vi "Init DFRobot_Gravity_GNSS.vi"(8 "error in (no error)":errorcluster, 11 "DFRobot_Gravity_GNSS in":refnum<class "DFRobot_Gravity_GNSS.lvclass">) -> (0 "error out":errorcluster, 3 "DFRobot_Gravity_GNSS out":refnum<class "DFRobot_Gravity_GNSS.lvclass">)   [LabVIEW 2020, in "CTI-Peripheral.lvlib" / "DFRobot_Gravity_GNSS.lvclass"]
uses:
  DFRobot_Gravity_GNSS.lvclass
  GPSData.ctl
  Power.ctl
  eGnssMode.ctl
  DFRobot_Gravity_GNSS.lvclass/DFRobot_Gravity_GNSS.ctl
  CTI/I2C Connection/I2C Connection.lvclass/I2C Connection.ctl
  CTI/Session/I2C Write Data.vi
  CTI/I2C Connection/I2C Connection.lvclass
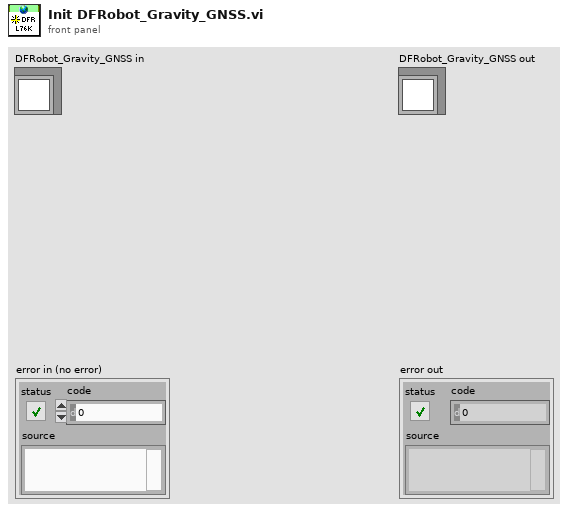
[diagram p1: front panel]
types:
  T1 = typedef "CTI-Peripheral.lvlib/DFRobot_Gravity_GNSS.lvclass/eGnssMode.ctl" = enum16{"No Mode - Error", "eGPS", "eBeiDou", "eGPS_BeiDou", "eGLONASS", "eGPS_eGLONASS", "eGPS_BeiDou_GLONASS"}
  T2 = typedef "CTI-Peripheral.lvlib/DFRobot_Gravity_GNSS.lvclass/GPSData.ctl" = u16
  T3 = typedef "CTI-Peripheral.lvlib/DFRobot_Gravity_GNSS.lvclass/Power.ctl" = enum16{"Enable", "Disable"}
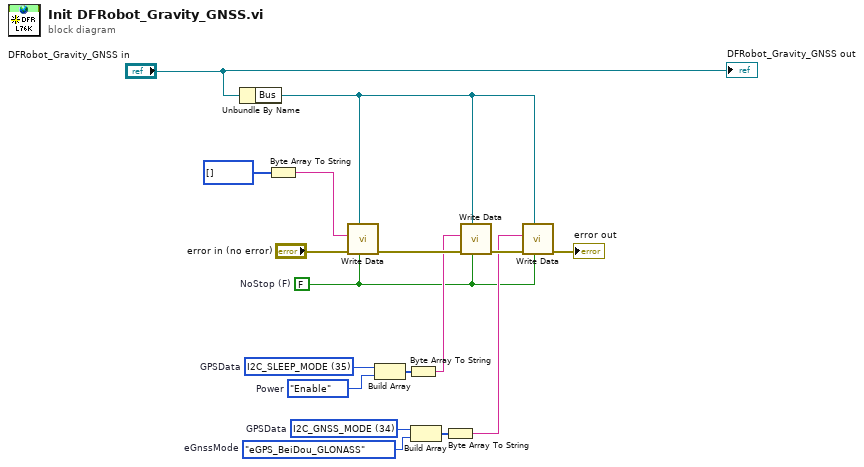
[diagram p0: block diagram]
diagram:
  w2 = eGnssMode."eGPS_BeiDou_GLONASS"  # eGnssMode
  w3 = T2 34 items=["I2C_YEAR_H", "I2C_YEAR_L", "I2C_MONTH", "I2C_DATE", "I2C_HOUR", "I2C_MINUTE", "I2C_SECOND", "I2C_LAT_1", "I2C_LAT_2", "I2C_LAT_X_24", "I2C_LAT_X_16", "I2C_LAT_X_8", "I2C_LON_DIS", "I2C_LON_1", "I2C_LON_2", "I2C_LON_X_24", "I2C_LON_X_16", "I2C_LON_X_8", "I2C_LAT_DIS", "I2C_USE_STAR", "I2C_ALT_H", "I2C_ALT_L", "I2C_ALT_X", "I2C_SOG_H", "I2C_SOG_L", "I2C_SOG_X", "I2C_COG_H", "I2C_COG_L", "I2C_COG_X", "I2C_START_GET", "I2C_ID", "I2C_DATA_LEN_H", "I2C_DATA_LEN_L", "I2C_ALL_DATA", "I2C_GNSS_MODE", "I2C_SLEEP_MODE", "I2C_RGB_MODE"]  # GPSData
  w5 = Power."Enable"  # Power
  w6 = T2 35 items=["I2C_YEAR_H", "I2C_YEAR_L", "I2C_MONTH", "I2C_DATE", "I2C_HOUR", "I2C_MINUTE", "I2C_SECOND", "I2C_LAT_1", "I2C_LAT_2", "I2C_LAT_X_24", "I2C_LAT_X_16", "I2C_LAT_X_8", "I2C_LON_DIS", "I2C_LON_1", "I2C_LON_2", "I2C_LON_X_24", "I2C_LON_X_16", "I2C_LON_X_8", "I2C_LAT_DIS", "I2C_USE_STAR", "I2C_ALT_H", "I2C_ALT_L", "I2C_ALT_X", "I2C_SOG_H", "I2C_SOG_L", "I2C_SOG_X", "I2C_COG_H", "I2C_COG_L", "I2C_COG_X", "I2C_START_GET", "I2C_ID", "I2C_DATA_LEN_H", "I2C_DATA_LEN_L", "I2C_ALL_DATA", "I2C_GNSS_MODE", "I2C_SLEEP_MODE", "I2C_RGB_MODE"]  # GPSData
  w9 = FALSE  # NoStop (F)
  n1 = Unbundle By Name("DFRobot_Gravity_GNSS in") -> ("Bus"=w10:refnum<class "I2C Connection.lvclass">)
  n2 = Byte Array To String(unsigned byte array=u8[] []) -> (string=w15:string)
  n3 = call "Write Data.vi"("NoStop (F)"=w9, "I2C Connection"=w10, "error in (no error)"="error in (no error)", "Data"=w15) -> ("error out"=w14:errorcluster)  [unwired: 7 in]
  n4 = Build Array(w6, w5) -> (w16:T2[])
  n5 = Byte Array To String(unsigned byte array=w16) -> (string=w13:string)
  n6 = Build Array(w3, w2) -> (w1:T2[])
  n7 = Byte Array To String(unsigned byte array=w1) -> (string=w11:string)
  n8 = call "Write Data.vi"("NoStop (F)"=w9, "I2C Connection"=w10, "error in (no error)"=w14, "Data"=w13) -> ("error out"=w12:errorcluster)  [unwired: 7 in]
  n9 = call "Write Data.vi"("NoStop (F)"=w9, "I2C Connection"=w10, "error in (no error)"=w12, "Data"=w11) -> ("error out"=→"error out":errorcluster)  [unwired: 7 in]
  "DFRobot_Gravity_GNSS out" <- "DFRobot_Gravity_GNSS in"
